vi "Avoid Shooter Death.vi"(6 "Shooter Angle":dbl, 10 "Proposed Power":dbl, 11 "CAN Talon SRX Ref":T1={"DeviceStatus"={"status"=FALSE, "code"=0, "source"=""}, "Type"=enum."PWM", "PWM"={"PWM Channel"=enum."PWM 1", "DeadBand"={"Name"="", "maxPositivePwm"=0, "minPositivePwm"=0, "centerPwm"=0, "maxNegativePwm"=0, "minNegativePwm"=0, "angularRange"=0}}, "CAN"={"Device Number"=0, "Control Mode"=enum."Percent VBus", "Semaphore"=refnum, "Max Vout"=12.0, "TalonSRX Control Mode"=enum."Percent VBus"}, "Invert"=FALSE}) -> (0 "Reverse Trip?":bool, 1 "Forward Trip?":bool, 2 "Actual Output":dbl, 3 "CAN Talon SRX Ref 2":T1={"DeviceStatus"={"status"=FALSE, "code"=0, "source"=""}, "Type"=enum."PWM", "PWM"={"PWM Channel"=enum."PWM 1", "DeadBand"={"Name"="", "maxPositivePwm"=0, "minPositivePwm"=0, "centerPwm"=0, "maxNegativePwm"=0, "minNegativePwm"=0, "angularRange"=0}}, "CAN"={"Device Number"=0, "Control Mode"=enum."Percent VBus", "Semaphore"=refnum, "Max Vout"=12.0, "TalonSRX Control Mode"=enum."Percent VBus"}, "Invert"=FALSE})   [LabVIEW 2015]
uses:
  Robot Global Data.vi
  Common Code/Change Detect Boolean.vi
  <vilib>/Rock Robotics/WPI/CAN/Jaguar/SubVIs/WPI_CANJaguar_ControlMode.ctl
  <vilib>/Rock Robotics/WPI/CAN/TalonSRX/WPI_CANTalonSRX_APIControlMode.ctl
  <vilib>/Rock Robotics/SystemInterfaces/DIO/FPGA_DIOPWMChannel.ctl
  <vilib>/Rock Robotics/WPI/PWM/WPI_PWMDeadband.ctl
  <vilib>/Rock Robotics/WPI/MotorControl/WPI_MotorControlType.ctl
  <vilib>/Rock Robotics/WPI/MotorControl/WPI_MotorControlDeviceRef.ctl
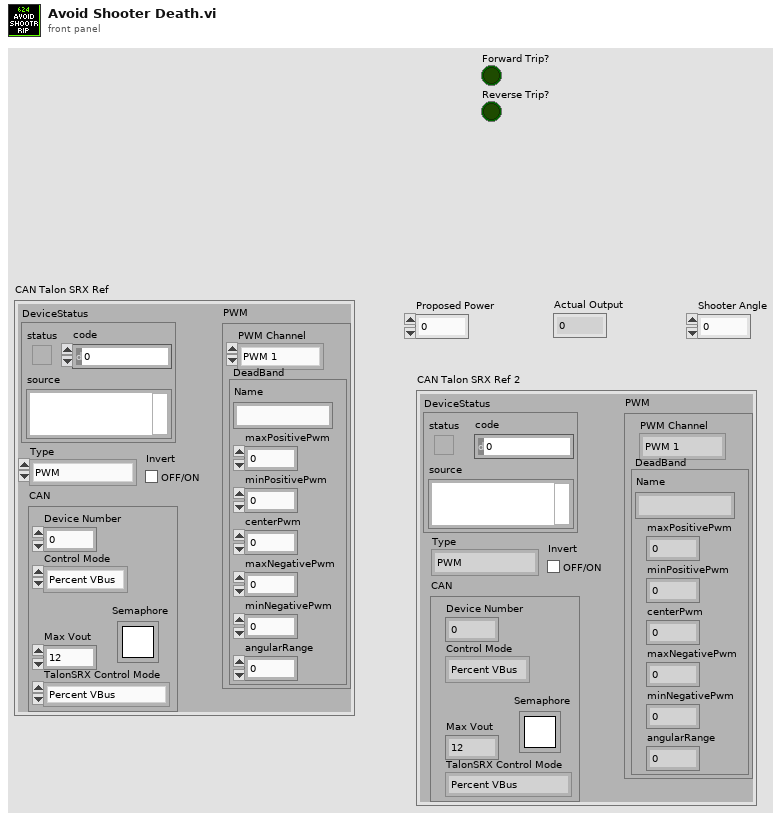
[diagram p1: front panel]
types:
  T1 = typedef "WPI_MotorControlDeviceRef.ctl" = cluster{"DeviceStatus":errorcluster, "Type":T2, "PWM":cluster{"PWM Channel":T3, "DeadBand":T4}, "CAN":cluster{"Device Number":u8, "Control Mode":T5, "Semaphore":T6, "Max Vout":dbl, "TalonSRX Control Mode":T7}, "Invert":bool}
  T2 = typedef "WPI_MotorControlType.ctl" = enum16{"PWM", "CAN", "CANTalonSRX"}
  T3 = typedef "FPGA_DIOPWMChannel.ctl" = enum8{"PWM 0", "PWM 1", "PWM 2", "PWM 3", "PWM 4", "PWM 5", "PWM 6", "PWM 7", "PWM 8", "PWM 9", "PWM MXP 0", "PWM MXP 1", "PWM MXP 2", "PWM MXP 3", "PWM MXP 4", "PWM MXP 5", "PWM MXP 6", "PWM MXP 7", "PWM MXP 8", "PWM MXP 9", "Invalid"}
  T4 = typedef "WPI_PWMDeadband.ctl" = cluster{"Name":string, "maxPositivePwm":i32, "minPositivePwm":i32, "centerPwm":i32, "maxNegativePwm":i32, "minNegativePwm":i32, "angularRange":u16}
  T5 = typedef "WPI_CANJaguar_ControlMode.ctl" = enum8{"Percent VBus", "Current", "Speed", "Position", "Voltage"}
  T6 = typedef "Semaphore RefNum" = refnum<k1>
  T7 = typedef "WPI_CANTalonSRX_APIControlMode.ctl" = enum8{"Percent VBus", "Speed", "Position", "Slave", "Unchanged / Invalid", "Voltage Compensation", "Current", "Motion Profile"}
  T8 = typedef "Dashboard Control Data.ctl" = cluster{"Shooter Presets":T9, "Encoder Control":T11, "Steer PID output":cluster{"output high":dbl, "output low":dbl}, " Steer PID gains":cluster{"proportional gain (Kc)":dbl, "integral time (Ti, min)":dbl, "derivative time (Td, min)":dbl}, "Drivetrain Settings":T12, "Vision Packet":T13, "Dashboard Drivetrain Command":T14, "Info/Command Cluster":T16, "Ball Vision Packet":T17, "Intake Presets":T19, "Intake Encoder Control":T21, "Climb Presets":T22, "Goal Output Range":cluster{"output high":dbl, "output low":dbl}, "Enabled Systems":T23, "Auton Presets":T24, "Pressure M":dbl, "Pressure B":dbl, "Vision Timeout":dbl, "Auto-Shift":T25, "Catapult Setpoints":T26}
  T9 = typedef "Shooter Presets.ctl" = cluster{"Batter Shot":T10, "Deep Middle":T10, "Manual Shot":T10, "Left Ticks Per Rotation":dbl, "Right Ticks Per Rotation":dbl, "Low Bar Shot":T10, "Shooter RPM Tolerance":dbl, "Trigger Power":dbl, "Fire from Load Delay":i32, "Max Angle":dbl, "Min Angle":dbl, "Angle PID gains":cluster{"P":dbl, "I":dbl, "D":dbl}, "Angle Output":cluster{"output high":dbl, "output low":dbl}, "Shooter Angle Tolerance":dbl, "Vision Shoot x^2":dbl, "Vision Shoot x":dbl, "Feed Forward Max Accel":dbl, "Feed Forward Kv":dbl, "Backwards Trigger":dbl, "Shot Finish Delay (ms)":dbl, "Angle Max Current":dbl, "Angle Current Trip Time":dbl, "Intake Angle":dbl, "Vision Shoot c":dbl, "Reset?":bool, "Button Release Delay":dbl, "Angle Pot x":dbl, "Angle Pot c":dbl, "Ignore Angle?":bool, "Max RPM":dbl, "Safty Frist Angle":dbl, "Intake Danger Height":dbl, "Angle Pot B":i32, "Angle Pot M":dbl, "FF Finish RPM":dbl, "RPM PID Right":cluster{"P":dbl, "I":dbl, "D":dbl, "FF":dbl}, "RPM PID Left":cluster{"P":dbl, "I":dbl, "D":dbl, "FF":dbl}, "Backwards RPM":dbl, "Vision RPM":dbl, "Run Wheels Backward Delay":u32, "Cleat Shot":T10, "Vision Far RPM":dbl, "Vision Far Distance":dbl, "Vision Far Angle":dbl}
  T10 = typedef "Shot Presets.ctl" = cluster{"L":dbl, "R":dbl, "A":dbl}
  T11 = typedef "Encoder Control.ctl" = cluster{"Right Tick Constant":dbl, "Left Tick Constant":dbl, "Reset?":bool, "Y Dist":cluster{"PID gains":cluster{"proportional gain (Kc)":dbl, "integral time (Ti, min)":dbl, "derivative time (Td, min)":dbl}}, "Y Stop Thresh":dbl, "Y Stop Speed":dbl}
  T12 = typedef "Drivetrain Settings.ctl" = cluster{"Gyro Tolerance":dbl, "Throttle Ramp (ms)":dbl, "Kv":dbl, "Ka":dbl, "Feed Forward P":dbl, "Feed Forward D":dbl, "Goal Vision PID gains":cluster{"proportional gain (Kc)":dbl, "integral time (Ti, min)":dbl, "derivative time (Td, min)":dbl}, "Goal Detection Window":dbl, "Creep Rate":dbl, "Vision Throttle Threshold":dbl, "Min Turn Output":dbl, "Left Batter Angle":dbl, "Right Batter Angle":dbl}
  T13 = typedef "Goal Vision Packet.ctl" = cluster{"Distance":dbl, "Center X":dbl, "Center Y":dbl, "Found Target?":bool, "Robot Center":dbl, "Angle":dbl}
  T14 = typedef "Dashboard Drivetrain Command.ctl" = cluster{"Drivetrain Vision":T15}
  T15 = typedef "Drivetrain Vision.ctl" = cluster{"Goal Window":dbl, "Ball Window":dbl}
  T16 = typedef "Ball Tracking Command Cluster.ctl" = cluster{"Distance to Ball":dbl, "Desired Angle":dbl, "Command":enum16{"Turn to Ball", "Turn to Angle", "Get Distance"}, "Pixels from Center":dbl}
  T17 = typedef "Ball Vision Packet.ctl" = cluster{"Ball Detected?":bool, "Distance to Ball":dbl, "Desired Angle":dbl, "Pixels from Center":dbl, "Tracking mode":T18}
  T18 = typedef "Tracking Mode.ctl" = enum16{"Turn to Ball", "Turn to Angle"}
  T19 = typedef "Intake Presets.ctl" = cluster{"Intake Speed":dbl, "Outake Speed":dbl, "Low Height":dbl, "Half Height":dbl, "High Idle Height":dbl, "Angle Speed":dbl, "Angle Tolerance":dbl, "Encoder Scale":dbl, "Load Height":dbl, "Output Range":T20, "Rotation Power Max/Min":dbl, "MaxCurrent":dbl, "Intake Trip Time":dbl, "Idle Height":dbl, "Max Height":dbl, "Reset Encoders?":bool, "PID gains":cluster{"proportional gain (Kc)":dbl, "integral time (Ti, min)":dbl, "derivative time (Td, min)":dbl}, "Intake Stop Delay":u32, "Settle Time":dbl, "Settle Wait Time":dbl, "Pull Up Delay":dbl}
  T20 = typedef "Drivetrain Output Range.ctl" = cluster{"output high":dbl, "output low":dbl}
  T21 = typedef "IntakeEcoderControl.ctl" = cluster{"Arm Tick Constant":dbl, "Reset?":bool, "Y Dist":cluster{"PID gains":cluster{"proportional gain (Kc)":dbl, "integral time (Ti, min)":dbl, "derivative time (Td, min)":dbl}}, "Y Stop Thresh":dbl, "Y Stop Speed":dbl}
  T22 = typedef "Climb Presets.ctl" = cluster{"Pull Power":dbl, "Extend Power":dbl}
  T23 = typedef "Enabled Systems.ctl" = cluster{"Shoot":bool, "Intake":bool, "DT":bool, "Gyro":bool, "100ms":bool, "US":bool}
  T24 = typedef "Autonomous Presets.ctl" = cluster{"Pitch Limit":dbl, "Roll Limit":dbl, "Start Position":dbl, "Cross Position":dbl}
  T25 = typedef "Auto Shift Cluster.ctl" = cluster{"Delay":dbl, "Speed Thresh":dbl, "Upshift Accel":dbl, "Upshift Throttle":dbl, "Upshift Throttle Accel":dbl, "Downshift Throttle":dbl, "Downshift Throttle Accel":dbl, "Pressure Threshold":dbl}
  T26 = typedef "Catapult Setpoints.ctl" = cluster{"Intake Danger Height":dbl, "Claw Release Delay":dbl}
  T27 = typedef "WPI_CANTalonSRX_GlobalStatus.ctl" = cluster{"Applied Throttle":dbl, "Module Enabled":bool, "CAN Error":errorcluster, "Closed Loop Error":dbl, "Forward Limit Switch Closed":bool, "Reverse Limit Switch Closed":bool, "Sensor Position":dbl, "Sensor Velocity":dbl, "Current":dbl, "Sticky Fault - Over Temp":bool, "Sticky Fault - Under Voltage":bool, "Sticky Fault - Forward Limit":bool, "Sticky Fault - Reverse Limit":bool, "Sticky Fault - Forward Soft Limit":bool, "Sticky Fault - Reverse Soft Limit":bool, "Brake is Enabled":bool, "Encoder Position":dbl, "Encoder Velocity":dbl, "Encoder Index Count":dbl, "Encoder A Pin State":bool, "Encoder B Pin State":bool, "Encoder Index Pin State":bool, "Analog In":dbl, "Analog In Velocity":dbl, "Temperature (C)":dbl, "Battery Voltage":dbl, "Control 5 Is Supported":bool, "Current Profile Slot Select":dbl, "Pos Div 8":bool, "Vel Div 4":bool, "Pulse Width Position":i32, "Pulse Width Velocity":i32, "Pulse Width Rise To Rise (us)":i32, "Pulse Width Rise To Fall (us)":i32, "Mot Prof Active Is Under Run":bool, "Mot Prof Active Has Under Run":bool, "Mot Prof Active Is Last":bool, "Mot Prof Active Velocity Only":bool, "Mot Prof Active Is Valid":bool, "Mot Prof Buffer Is Full":bool, "Mot Prof Active Profile Slot Select":i32, "Mot Prof NextID":i32, "Mot Prof Count":i32, "Mot Prof Active Velocity":dbl, "Mot Prof Active Position":dbl, "Mot Prof Output Enable":i32}
  T28 = typedef "WPI_DriverStationRobotMode2.ctl" = enum16{"Autonomous Disabled", "Autonomous Enabled", "Teleop Disabled", "Teleop Enabled", "Disconnected", "Finish", "Test Disabled", "Test Enabled", "Emergency Stopped"}
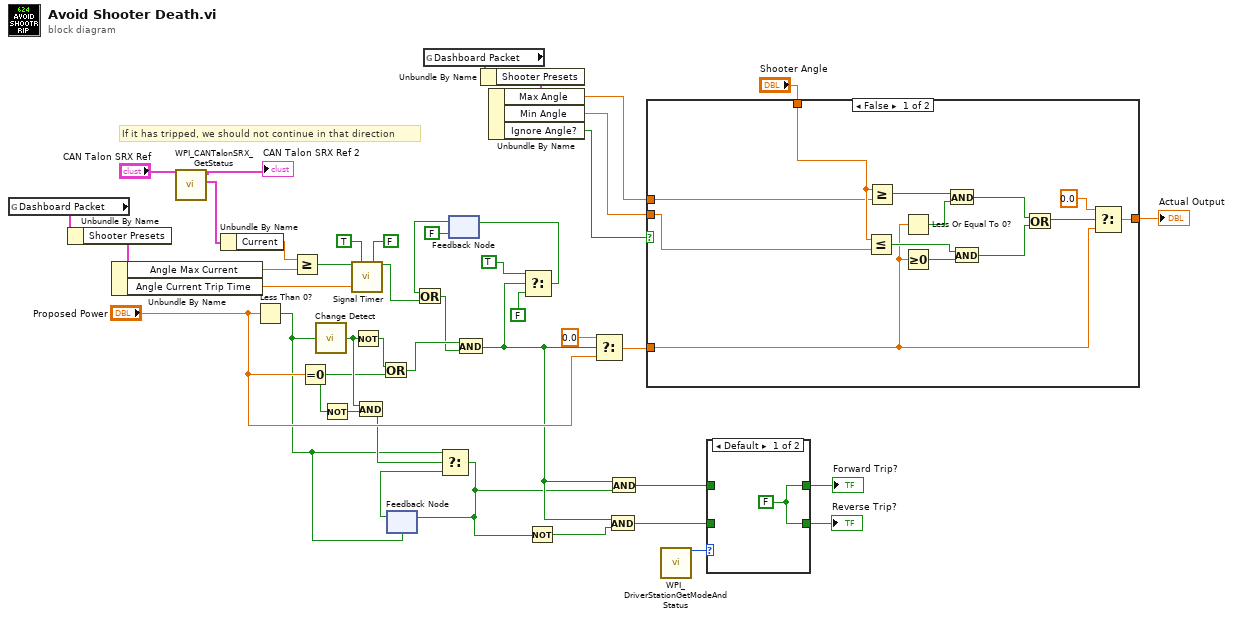
[diagram p0: block diagram]
diagram:
  # "If it has tripped, we should not continue in that direction"
  n1 = global read "Robot Global Data.vi" "Dashboard Packet"() -> (w44:T8)
  n2 = Unbundle By Name(w44) -> ("Shooter Presets"=w43:T9)
  n3 = Unbundle By Name(w43) -> ("Angle Max Current"=w42:dbl, "Angle Current Trip Time"=w38:dbl)
  n4 = call <vilib>:"WPI_CANTalonSRX_GetStatus.vi"("CAN Talon SRX Ref"="CAN Talon SRX Ref") -> ("Talon SRX Status"=w9:T27, "CAN Talon SRX Ref"=→"CAN Talon SRX Ref 2":T1)  [unwired: 8 in, 1 out]
  n5 = Unbundle By Name(w9) -> ("Current"=w8:dbl)
  n6 = Less Than 0?(x="Proposed Power") -> (x < 0?=w18:bool)
  n7 = Greater Or Equal?(x=w8, y=w42) -> (x >= y?=w41:bool)
  n8 = Equal To 0?(x="Proposed Power") -> (x = 0?=w24:bool)
  n9 = call-poly "Change Detect.vi"("In"=w18) -> ("Changed?"=w25:bool)
  n10 = Not(x=w24) -> (.not. x?=w23:bool)
  n11 = call "Signal Timer.vi"("Input"=w41, "Edge"=TRUE, "Interval"=w38, "Pull"=FALSE) -> ("Filtered Output"=w33:bool)  [unwired: 11 in]
  n12 = Not(x=w25) -> (.not. x?=w37:bool)
  n13 = And(x=w25, y=w23) -> (x .and. y?=w22:bool)
  n14 = Or(x=w37, y=w24) -> (x .or. y?=w36:bool)
  n15 = feedback #1(w18) -> (w21:bool)
  n16 = global read "Robot Global Data.vi" "Dashboard Packet"() -> (w14:T8)
  n17 = Select(t=w18, s=w22, f=w21) -> (s? t:f=w20:bool)
  n18 = feedback-in #1(w20) -> ()
  n19 = feedback #2(FALSE) -> (w30:bool)
  n20 = Or(x=w30, y=w33) -> (x .or. y?=w32:bool)
  n21 = And(x=w36, y=w32) -> (x .and. y?=w26:bool)
  n22 = Unbundle By Name(w14) -> ("Shooter Presets"=w13:T9)
  n23 = Unbundle By Name(w13) -> ("Max Angle"=w12:dbl, "Min Angle"=w11:dbl, "Ignore Angle?"=w10:bool)
  n24 = Select(t=TRUE, s=w26, f=FALSE) -> (s? t:f=w31:bool)
  n25 = feedback-in #2(w31) -> ()
  n26 = Not(x=w20) -> (.not. x?=w19:bool)
  n27 = Select(t=0.0, s=w26, f="Proposed Power") -> (s? t:f=w17:dbl)
  n28 = And(x=w26, y=w19) -> (x .and. y?=w5:bool)
  n29 = And(x=w26, y=w20) -> (x .and. y?=w3:bool)
  n30 = case shown="False" w10 {
    tunnel: w17 -> [w47 w58]
    tunnel: [w51 w58] -> w16
    tunnel: "Shooter Angle" -> [w50 _]
    tunnel: w12 -> [w49 _]
    tunnel: w11 -> [w48 _]
    frame False {
      n31 = Less Or Equal?(x=w50, y=w48) -> (x <= y?=w57:bool)
      n32 = Greater Or Equal?(x=w50, y=w49) -> (x >= y?=w56:bool)
      n33 = Less Or Equal To 0?(x=w47) -> (x <= 0?=w46:bool)
      n34 = Greater Or Equal To 0?(x=w47) -> (x >= 0?=w45:bool)
      n35 = And(x=w56, y=w46) -> (x .and. y?=w55:bool)
      n36 = And(x=w57, y=w45) -> (x .and. y?=w54:bool)
      n37 = Or(x=w55, y=w54) -> (x .or. y?=w53:bool)
      n38 = Select(t=0.0, s=w53, f=w47) -> (s? t:f=w51:dbl)
    }
    frame True {
    }
  }
  "Actual Output" <- w16
  n39 = call <vilib>:"WPI_DriverStationGetModeAndStatus.vi"() -> ("Robot Mode"=w7:T28)  [unwired: 10 in, 1 out]
  n40 = case shown="Default" w7 {
    tunnel: [w59 w61] -> w6
    tunnel: w5 -> [_ w61]
    tunnel: [w59 w60] -> w4
    tunnel: w3 -> [_ w60]
    frame Default {
      w59 = FALSE
    }
    frame "Autonomous Enabled", "Teleop Enabled" {
    }
  }
  "Forward Trip?" <- w4
  "Reverse Trip?" <- w6
